vi "Close.vi"(8 "error in (no error)":errorcluster caption="entrée d'erreur (pas d'erreur)", 11 "Class Printer_CAB en entrée":refnum<class "Class Printer_CAB.lvclass">) -> (0 "error out":errorcluster caption="sortie d'erreur", 3 "Class Printer_CAB en sortie":refnum<class "Class Printer_CAB.lvclass">)   [LabVIEW 2020, in "Library Instrument & Equipement.lvlib" / "Library Printer.lvlib" / "Class Printer_CAB.lvclass"]
uses:
  Class Printer_CAB.lvclass
  Class Printer_CAB.lvclass/Class Printer_CAB.ctl
  Printer (Default)/Class Printer (Default).lvclass
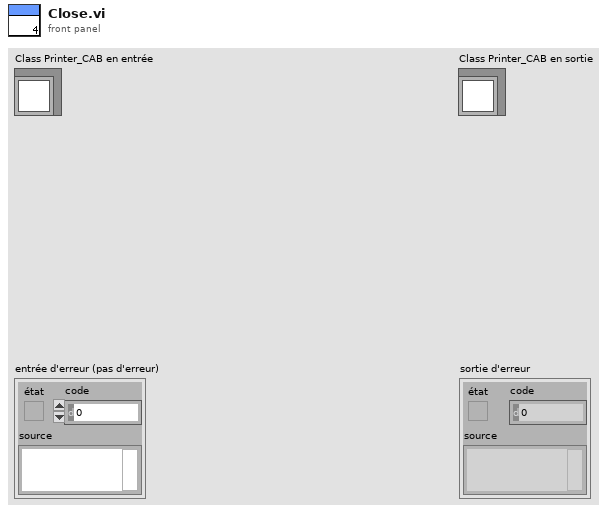
[diagram p1: front panel]
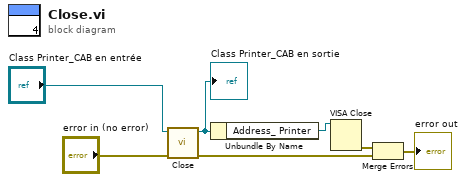
[diagram p0: block diagram]
diagram:
  n1 = call-parent "Close.vi"("error in (no error)"="error in (no error)", "Class Printer (Default) en entrée"="Class Printer_CAB en entrée") -> ("error out"=w3:errorcluster, "Class Printer (Default) en sortie"=w5:refnum<class "Class Printer_CAB.lvclass">)  [unwired: 8 in]
  "Class Printer_CAB en sortie" <- w5
  n2 = Unbundle By Name(w5) -> ("Address_ Printer"=w1:refnum<visa-resource-name>)
  n3 = VISA Close(VISA resource name=w1) -> (error out=w4:errorcluster)  [unwired: 1 in]
  n4 = Merge Errors(w4, w3) -> (→"error out":errorcluster)
